vi "Box_Create.vi"(0 "reference in":refnum<class "Box.lvclass">, 5 "Error In":errorcluster) -> (14 "reference out":refnum<class "Box.lvclass">, 19 "Error Out":errorcluster)   [LabVIEW 2024, in "Box.lvclass"]
uses:
  Box.lvclass/Box.ctl
  Box.lvclass
panel:
  # "Connector Pane"
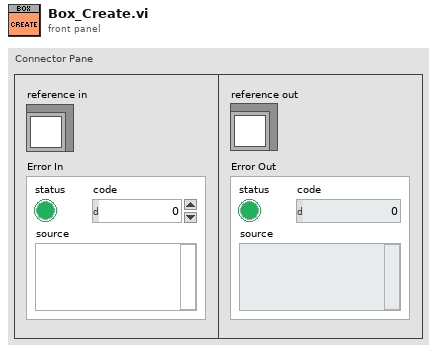
[diagram p1: front panel]
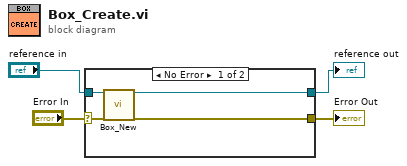
[diagram p0: block diagram]
diagram:
  n1 = case shown="No Error" "Error In" {
    selector: "Error In" -> [w7 w10]
    tunnel: [w5 w10] -> w3
    tunnel: "reference in" -> [w8 w9]
    tunnel: [w6 w9] -> w1
    frame No Error {
      n2 = call "Box_New.vi"("reference in"=w8, "Error In"=w7) -> ("reference out"=w6:refnum<class "Box.lvclass">, "Error Out"=w5:errorcluster)  [unwired: 14 in, 2 out]
    }
    frame Error {
      # "VI-TechBaseTemplate_Simple_6x8x6"
    }
  }
  "Error Out" <- w3
  "reference out" <- w1
